vi "EnvFloInit.vi"(8 "error in (no error)":errorcluster, 10 "db connection in":T1, 11 "VISA Refnum in":refnum<visa-resource-name>) -> (0 "error out":errorcluster, 1 "sensor id":i32, 2 "db connection out":T1, 3 "VISA Refnum out":refnum<visa-resource-name>)   [LabVIEW 2016]
uses:
  <vilib>/addons/database/Connection.llb/Conn ObjectReference.ctl
  <vilib>/addons/database/NI_Database_API.lvlib
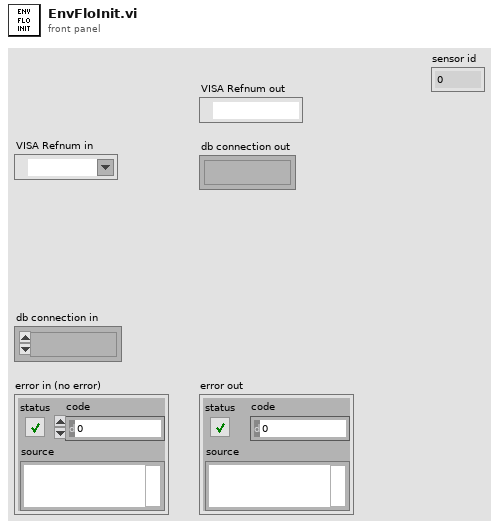
[diagram p1: front panel]
types:
  T1 = typedef "NI_Database_API.lvlib/Conn ObjectReference.ctl" = refnum<k1>
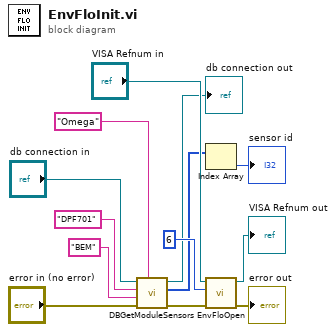
[diagram p0: block diagram]
diagram:
  n1 = call "DBGetModuleSensors.vi"("Module make"="Omega", "error in (no error)"="error in (no error)", "Module loc"="BEM", "Module model"="DPF701", "db connection in"="db connection in") -> ("error out"=w11:errorcluster, "sensor id array"=w2:i32[], "db connection out"=→"db connection out":T1)  [unwired: 3 in, 1 out]
  n2 = Index Array(array=w2) -> (element=→"sensor id":i32)  [unwired: 1 in]
  n3 = call "EnvFloOpen.vi"("error in (no error)"=w11, "read timeout"=u32 6, "VISA Refnum in"="VISA Refnum in") -> ("error out"=→"error out":errorcluster, "VISA Refnum out"=→"VISA Refnum out":refnum<visa-resource-name>)  [unwired: 7 in]
